vi "Term_Project_AM.vi"() -> ()   [LabVIEW 2012]
doc: "This VI illustrates how to perform simultaneous sound IO, i.e., how to continuously play the sound acquired from a microphone. It requires the use of a microphone attached to the sound card. You can specify the IDs of the input and output devices, the frequency to sample at, and the buffer size for both devices. Higher frequencies have better quality, but demand more resources and are limited by the capabilities of your sound card. A large number of samples decreases the risk of glitches, but increases the delay between acquisition and playback."
uses:
  <vilib>/sound2/lvsound2.llb/Sound Data Format.ctl
  <vilib>/sound2/lvsound2.llb/Sampling Mode.ctl
  <vilib>/Analysis/3filter.llb/Filter Passband Type.ctl
  <vilib>/sound2/lvsound2.llb/Sound Output Write (DBL Single).vi
  <instrlib>/niUSRP/niUSRP Write Tx Data (CDB).vi
  <instrlib>/niUSRP/niUSRP Fetch Rx Data (CDB WDT).vi
  <vilib>/measure/maspectr.llb/FFT Power Spectrum and PSD for 1 Chan.vi
  <vilib>/Analysis/3filter.llb/Butterworth Filter (DBL).vi
  <vilib>/sound2/lvsound2.llb/Sound Input Read (DBL).vi
  <vilib>/imath/engines/lvmath2/RunTimeEngine/NodeEndStatement/NIMS_NodeEndStatement_Output.vi
  <instcachedir>/0/NIMS_NodeEndStatement_Output_53EC0D466D134D7ABD903AC30B43404B.lvgen/NIMS_NodeEndStatement_Output_53EC0D466D134D7ABD903AC30B43404B_000.vi
  <instcachedir>/0/NIMS_NodeEndStatement_Output_53EC0D466D134D7ABD903AC30B43404B.lvgen/NIMS_NodeEndStatement_Output_53EC0D466D134D7ABD903AC30B43404B_005.vi
  <vilib>/imath/engines/lvmath2/RunTimeEngine/BuiltInFunctions/abs/NIMS_abs(signed).vi
  <instcachedir>/0/NIMS_abs(signed)_C4FCB8E6058B49B797C7C8D53CA5F6EC.lvgen/NIMS_abs(signed)_C4FCB8E6058B49B797C7C8D53CA5F6EC_001.vi
  <vilib>/imath/engines/lvmath2/RunTimeEngine/BuiltInFunctions/max/1 input/NIMS_max(RV).vi
  <instcachedir>/0/NIMS_max(RV)_237633DB1D604D5BA7001287DF3C7957.lvgen/NIMS_max(RV)_237633DB1D604D5BA7001287DF3C7957_000.vi
  <vilib>/imath/engines/lvmath2/RunTimeEngine/ErrorHandling/NIMS_Finalize Error.vi
  <vilib>/Analysis/NI_AALBase.lvlib
  <vilib>/measure/NI_MAPro.lvlib
panel:
  out "Press 2":bool
  in  "Press":bool
  out "Stop 2":bool
  in  "x":dbl=2.0
  in  "Output Device ID":u32
  out "error out":errorcluster
  out "Baseband Output":dbl[](graph)
  out "Power Spectrum":cluster{"f0":dbl, "df":dbl, "magnitude":dbl[]}(graph)
  out "Filtered X":dbl[](array[numeric])
  in  "active antenna":string="RX2"
  out "actual gain (dB)":dbl format="%#_6f"
  in  "gain (dB) (Rx)":dbl format="%#_6f"
  out "actual carrier frequency":dbl=100000.0 format="%#_6p"
  out "actual IQ rate (Rx)":dbl=100000.0 format="%#_6p"
  in  "IQ rate (Rx)":dbl=1000000.0 format="%#_6p"
  in  "device names":refnum<k15>="192.168.10.2"
  out "G":cdb[](array[numeric])
  in  "active antenna (Tx)":string="TX1"
  out "actual gain (dB) (Tx)":dbl format="%#_6f"
  in  "gain (dB) (Tx)":dbl format="%#_6f"
  out "actual carrier frequency (Tx)":dbl=100000.0 format="%#_6p"
  out "actual IQ rate (Tx)":dbl=100000.0 format="%#_6p"
  in  "IQ rate (Tx)":dbl=200000.0 format="%#_6p"
  in  "Tx device":refnum<k15>="192.168.10.2"
  in  "carrier frequency":u16(ring) items=["500 MHz", "300 MHz", "200 MHz"]
  out "Baseband Signal":dbl[](graph)
  out "Message":waveform(dbl)[](graph)
  in  "Modulation index":dbl(slide)=1.0 min=0.0 max=1.0 scale=0.0..1.0
  in  "Stop":bool
  in  "Input Device ID":u32
  # "TRANSMITTING"
  # "CONTROL"
  # "RECEIVING"
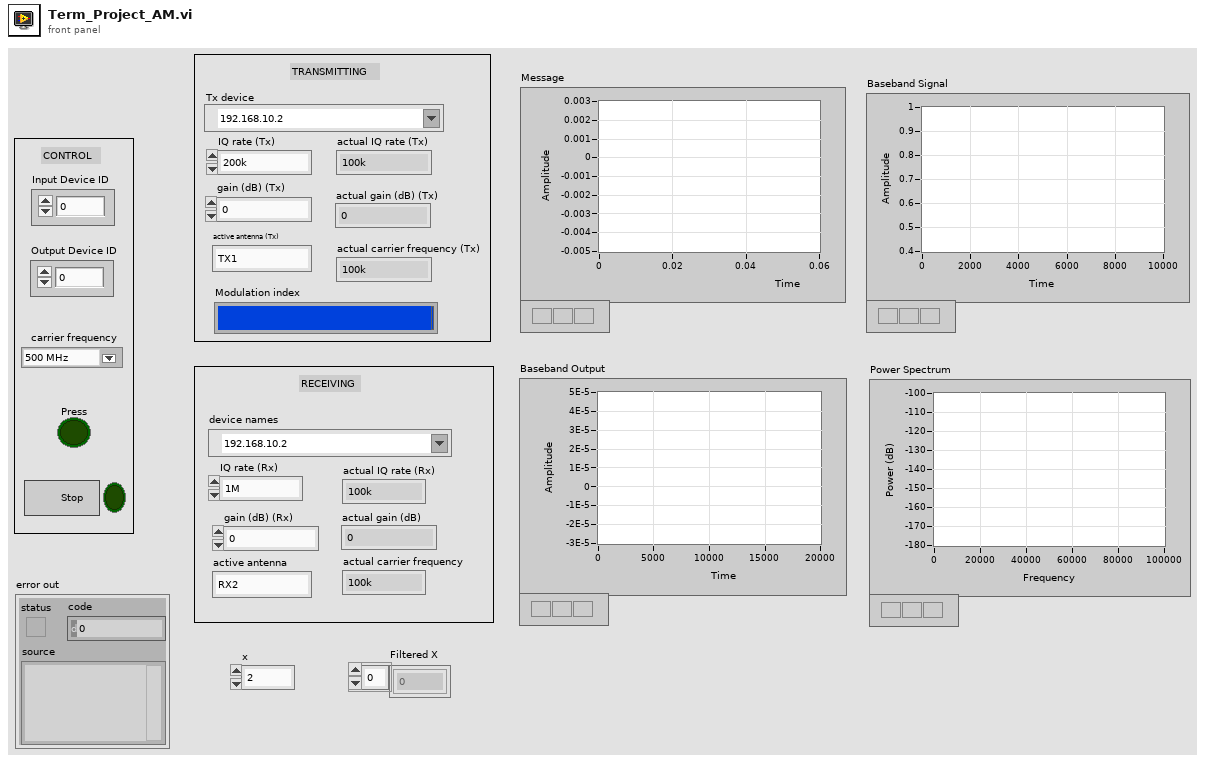
[diagram p1: front panel]
types:
  T1 = typedef "Sampling Mode.ctl" = i32
  T2 = typedef "Sound Data Format.ctl" = cluster{"sample rate (S/s)":dbl, "number of channels":i32, "bits per sample":i32}
  T3 = typedef "Sound Input Task ID.ctl" = u32
  T4 = typedef "Sound Output Task ID.ctl" = u32
  T5 = typedef "NI_AALBase.lvlib/Filter Passband Type.ctl" = enum32{"Lowpass", "Highpass", "Bandpass", "Bandstop"}
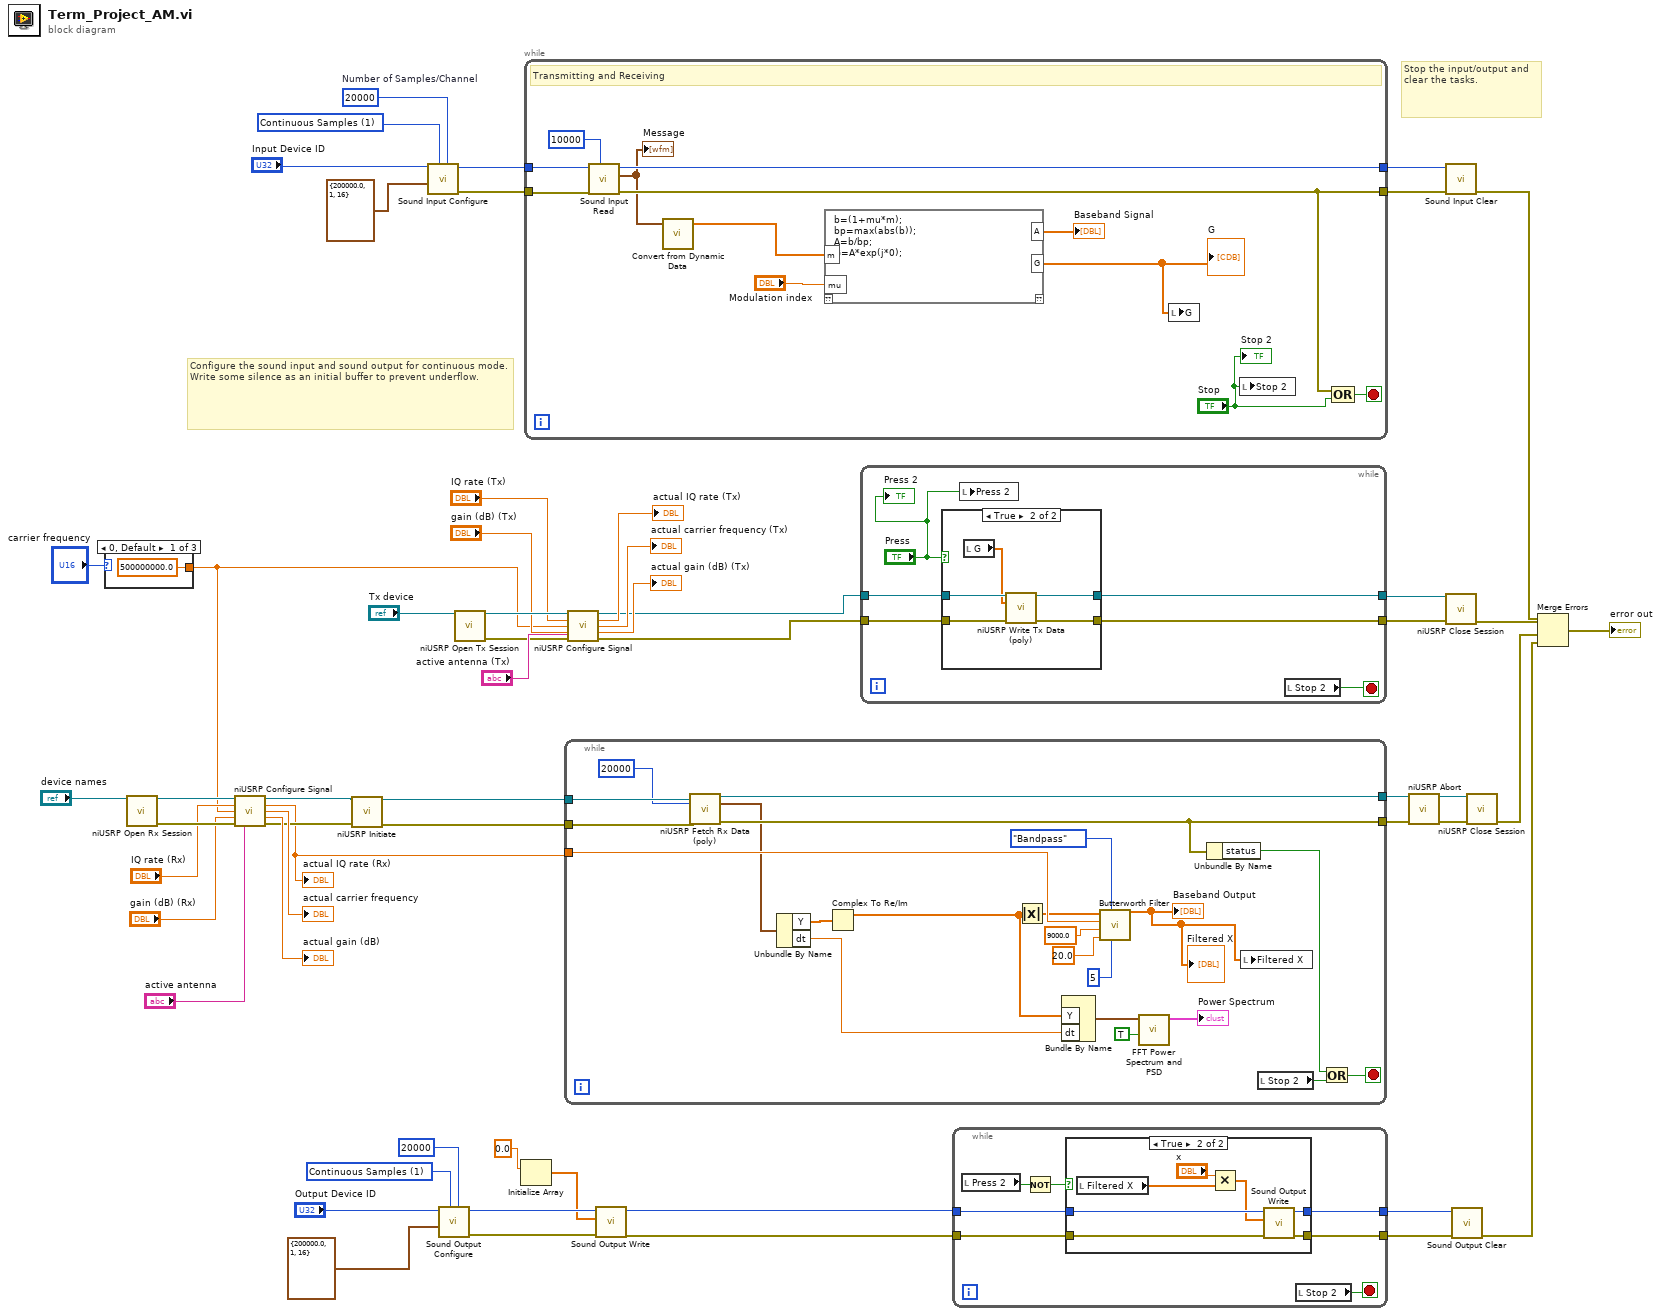
[diagram p0: block diagram]
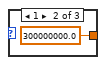
[diagram p4: hidden frame]
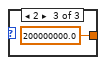
[diagram p5: hidden frame]
diagram:
  w13 = T1 1 items=["Finite Samples", "Continuous Samples"] ("sample mode")
  w49 = 20000  # Number of Samples/Channel
  w50 = T1 1 items=["Finite Samples", "Continuous Samples"] ("sample mode")
  # "Stop the input/output and clear the tasks."
  # "Configure the sound input and sound output for continuous mode. Write some silence as an initial buffer to prevent underflow."
  n1 = case shown="0, Default" "carrier frequency" {
    tunnel: [500000000.0 ("sample rate (S/s)") 300000000.0 ("sample rate (S/s)") 200000000.0 ("sample rate (S/s)")] -> w5
    frame 0, Default {
    }
    frame 1 {
    }
    frame 2 {
    }
  }
  n2 = call <instrlib>:"niUSRP Open Rx Session.vi"("device names"="device names") -> ("session handle out"=w34:refnum<k15>, "error out"=w33:errorcluster)  [unwired: 13 in]
  n3 = call <instrlib>:"niUSRP Configure Signal.vi"("session handle"=w34, "IQ rate"="IQ rate (Rx)", "carrier frequency"=w5, "gain"="gain (dB) (Rx)", "error in (no error)"=w33, "active antenna"="active antenna") -> ("session handle out"=w28:refnum<k15>, "coerced IQ rate"=w19:dbl, "coerced carrier frequency"=→"actual carrier frequency":dbl, "coerced gain"=→"actual gain (dB)":dbl, "error out"=w27:errorcluster)  [unwired: 5 in]
  "actual IQ rate (Rx)" <- w19
  n4 = call <instrlib>:"niUSRP Initiate.vi"("session handle"=w28, "error in (no error)"=w27) -> ("session handle out"=w25:refnum<k15>, "error out"=w24:errorcluster)  [unwired: 12 in]
  n5 = call <vilib>:"Sound Input Configure.vi"("number of samples/ch"=w49, "sample mode"=w50, "sound format"=T2 {"sample rate (S/s)"=200000.0, "number of channels"=1, "bits per sample"=16} ("Sound Format"), "device ID"="Input Device ID") -> ("error out"=w53:errorcluster, "task ID"=w52:T3)  [unwired: 6 in]
  n6 = call <vilib>:"Sound Output Configure.vi"("number of samples/ch"=20000, "sample mode"=w13, "sound format"=T2 {"sample rate (S/s)"=200000.0, "number of channels"=1, "bits per sample"=16} ("Sound Format"), "device ID"="Output Device ID") -> ("error out"=w16:errorcluster, "task ID"=w17:T4)  [unwired: 6 in]
  n7 = call <instrlib>:"niUSRP Open Tx Session.vi"("device names"="Tx device") -> ("session handle out"=w46:refnum<k15>, "error out"=w42:errorcluster)  [unwired: 13 in]
  n8 = Initialize Array(0.0 ("element")) -> (w14:dbl[])  [unwired: 1 in]
  n9 = while {
    tunnel: w52 -> [w70]
    tunnel: [w72] -> w55
    tunnel: w53 -> [w69]
    tunnel: [w65] -> w57
    stop <- w71 stop-if-true
    # "Transmitting and Receiving"
    n10 = call-poly <vilib>:"Sound Input Read.vi"("number of samples/ch"=10000, "error in (no error)"=w69, "task ID"=w70) -> ("error out"=w65:errorcluster, "data"=w61:waveform(dbl)[], "task ID out"=w72:T3)  [unwired: 6 in]
    "Message" <- w61
    n11 = call "Convert from Dynamic Data"("Dynamic Data Type"=w61) -> ("Array"=w64:dbl[])  [unwired: 3 in]
    n12 = mathscript code="b=(1+mu*m);\nbp=max(abs(b));\nA=b/bp;\nG=A*exp(j*0);"("m"=w64, "mu"="Modulation index") -> ("A"=→"Baseband Signal":dbl[], "G"=w63:cdb[])  [unwired: 1 in, 1 out]
    "G" <- w63
    n13 = local write "G"(w63) -> ()
    n14 = local write "Stop 2"("Stop") -> ()
    n15 = Compound Arithmetic op=OR(w65, "Stop") -> (w71:bool)
    "Stop 2" <- "Stop"
  }
  n16 = while {
    tunnel: w25 -> [w141]
    tunnel: w24 -> [w140]
    tunnel: [w139] -> w23
    tunnel: [w136] -> w22
    tunnel: w19 -> [w129]
    stop <- w138 stop-if-true
    n17 = call-poly <instrlib>:"niUSRP Fetch Rx Data (poly).vi"("session handle"=w141, "number of samples"=i64 20000, "error in (no error)"=w140) -> ("session handle out"=w139:refnum<k15>, "data"=w125:waveform(cdb), "error out"=w136:errorcluster)  [unwired: 9 in, 1 out]
    n18 = Unbundle By Name(w125) -> ("Y"=w132:cdb[], "dt"=w126:dbl)
    n19 = Complex To Re/Im(x + iy=w132) -> (x=w122:dbl[])  [unwired: 1 out]
    n20 = Absolute Value(x=w122) -> (abs(x)=w127:dbl[])
    n21 = Bundle By Name("Y"=w122, "dt"=w126) -> (w124:waveform(dbl))  [unwired: 1 in]
    n22 = call-poly <vilib>:"Butterworth Filter.vi"("order"=5, "filter type"=Filter_Passband_Type."Bandpass", "low cutoff freq: fl"=20.0, "high cutoff freq: fh"=9000.0, "sampling freq: fs"=w129, "X"=w127) -> ("Filtered X"=w121:dbl[])  [unwired: 2 in, 1 out]
    "Baseband Output" <- w121
    "Filtered X" <- w121
    n23 = call-poly <vilib>:"FFT Power Spectrum and PSD.vi"("dB On (F)"=TRUE, "time signal"=w124) -> ("Power Spectrum / PSD"=→"Power Spectrum":cluster{"f0":dbl, "df":dbl, "magnitude":dbl[]})  [unwired: 6 in, 3 out]
    n24 = Unbundle By Name(w136) -> ("status"=w137:bool)
    n25 = local write "Filtered X"(w121) -> ()
    n26 = local read "Stop 2"() -> (w120:bool)
    n27 = Or(x=w137, y=w120) -> (x .or. y?=w138:bool)
  }
  n28 = call <instrlib>:"niUSRP Configure Signal.vi"("session handle"=w46, "IQ rate"="IQ rate (Tx)", "carrier frequency"=w5, "gain"="gain (dB) (Tx)", "error in (no error)"=w42, "active antenna"="active antenna (Tx)") -> ("session handle out"=w37:refnum<k15>, "coerced IQ rate"=→"actual IQ rate (Tx)":dbl, "coerced carrier frequency"=→"actual carrier frequency (Tx)":dbl, "coerced gain"=→"actual gain (dB) (Tx)":dbl, "error out"=w36:errorcluster)  [unwired: 5 in]
  n29 = call-poly <vilib>:"Sound Output Write.vi"("error in (no error)"=w16, "data"=w14, "task ID"=w17) -> ("error out"=w1:errorcluster, "task ID out"=w2:T4)  [unwired: 7 in]
  n30 = while {
    tunnel: w37 -> [w147]
    tunnel: [w146] -> w10
    tunnel: [w145] -> w11
    tunnel: w36 -> [w144]
    stop <- w143 stop-if-true
    n31 = case shown="True" "Press" {
      tunnel: w147 -> [w149 w154]
      tunnel: [w149 w153] -> w146
      tunnel: [w148 w152] -> w145
      tunnel: w144 -> [w148 w151]
      frame False {
      }
      frame True {
        n32 = local read "G"() -> (w150:cdb[])
        n33 = call-poly <instrlib>:"niUSRP Write Tx Data (poly).vi"("session handle"=w154, "data"=w150, "error in (no error)"=w151) -> ("session handle out"=w153:refnum<k15>, "error out"=w152:errorcluster)  [unwired: 11 in]
      }
    }
    n34 = local write "Press 2"("Press") -> ()
    n35 = local read "Stop 2"() -> (w143:bool)
    "Press 2" <- "Press"
  }
  n36 = while {
    tunnel: [w161] -> w3
    tunnel: [w160] -> w4
    tunnel: w2 -> [w159]
    tunnel: w1 -> [w158]
    stop <- w157 stop-if-true
    n37 = local read "Press 2"() -> (w156:bool)
    n38 = Not(x=w156) -> (.not. x?=w155:bool)
    n39 = case shown="True" w155 {
      tunnel: [w163 w170] -> w161
      tunnel: [w162 w169] -> w160
      tunnel: w159 -> [w163 w168]
      tunnel: w158 -> [w162 w167]
      frame False {
      }
      frame True {
        n40 = local read "Filtered X"() -> (w165:dbl[])
        n41 = Multiply(x="x", y=w165) -> (x*y=w164:dbl[])
        n42 = call-poly <vilib>:"Sound Output Write.vi"("error in (no error)"=w167, "data"=w164, "task ID"=w168) -> ("error out"=w169:errorcluster, "task ID out"=w170:T4)  [unwired: 7 in]
      }
    }
    n43 = local read "Stop 2"() -> (w157:bool)
  }
  n44 = call <instrlib>:"niUSRP Abort.vi"("session handle"=w23, "error in (no error)"=w22) -> ("session handle out"=w21:refnum<k15>, "error out"=w20:errorcluster)  [unwired: 12 in]
  n45 = call <vilib>:"Sound Input Clear.vi"("error in (no error)"=w57, "task ID"=w55) -> ("error out"=w54:errorcluster)  [unwired: 9 in]
  n46 = call <instrlib>:"niUSRP Close Session.vi"("session handle"=w10, "error in (no error)"=w11) -> ("error out"=w48:errorcluster)  [unwired: 13 in]
  n47 = call <vilib>:"Sound Output Clear.vi"("error in (no error)"=w4, "task ID"=w3) -> ("error out"=w7:errorcluster)  [unwired: 9 in]
  n48 = call <instrlib>:"niUSRP Close Session.vi"("session handle"=w21, "error in (no error)"=w20) -> ("error out"=w8:errorcluster)  [unwired: 13 in]
  n49 = Merge Errors(w54, w48, w8, w7) -> (→"error out":errorcluster)
